vi "Autonomous Independent.vi"   [LabVIEW 2014]
doc: "This VI is called when autonomous begins, and will automatically be terminated when autonomous ends. You can carry out timed or sensor driven robot movement independently without needing to return to the caller."
uses:
  <vilib>/Rock Robotics/Network Tables/SD Read Number.vi
  Global Variables/Refnum Names.vi
panel:
  # "Be sure to right-click and choose Data Operations>>Make Current Value default if you want to save the array values with the VI"
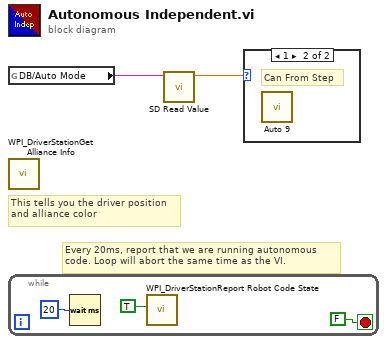
[diagram p0: block diagram]
diagram:
  # "Every 20ms, report that we are running autonomous\ncode. Loop will abort the same time as the VI."
  # "This tells you the driver position\nand alliance color"
  n1 = global read "Refnum Names.vi" "DB/Auto Mode"() -> (w1:string)
  n2 = call <vilib>:"WPI_DriverStationGet Alliance Info.vi"() -> ()  [unwired: 12 out]
  n3 = while {
    stop <- FALSE stop-if-true
    n4 = Wait (ms)(milliseconds to wait=u32 20) -> ()  [unwired: 1 out]
    n5 = call <vilib>:"WPI_DriverStationReport Robot Code State.vi"("Autonomous"=TRUE) -> ()  [unwired: 10 in, 1 out]
  }
  n6 = call-poly <vilib>:"SD Read Value.vi"("Name"=w1) -> ("Numeric"=w2:dbl)  [unwired: 8 in, 2 out]
  n7 = case shown="1" w2 {
    frame 0, Default {
      # "No Auto"
    }
    frame 1 {
      # "Can From Step"
      n8 = call "Auto 9.vi"() -> ()  [unwired: 11 in, 1 out]
    }
  }
